vi "RES Build RES Table.vi"(8 "error in (no error)":errorcluster, 9 "Test Types 2":refnum<vi>, 10 "Message Queues in":T1, 11 "Settings in":T2={"Support"={"Save Configuration"={"Log File Base Path"=path "", "TDMS File Reference"=refnum, "Reset"=FALSE, "Wait"=0.0, "Start Time"=0.0, "Update Rate"=0, "Channel Names"=[], "System Preset"=variant}, "LOG Configuration"={"LOG REF"=refnum, "Writer Queue"=refnum, "Log Path"=path "", "LOG"=FALSE}, "ALARM Configuration"={"LOG REF"=refnum, "Writer Queue"=refnum, "Log Path"=path "", "UPS standby"=FALSE, "status code"=0, "SP"=[], "Over Sens Status"=[]}, "User Details"=[], "Radome Type"="", "Timer Configuration"={"Wait"=0.0, "Next Step"="", "Writer Queue"=refnum, "Reset"=FALSE, "VISA resource"="", "Status"=[], "Valve Time"=[], "Timer queue"=refnum, "Current valve"=0, "Enable"=FALSE}}, "Process"={"Test Configuration"={"current Step"=0, "Wait"=0.0, "Next Step"="", "Writer Queue"=refnum, "Reset"=FALSE, "SEQ Time"=0, "General Reset"=FALSE, "Cycles"=0, "Status"=[], "Ready"=[], "Backward"=FALSE, "Current SP"=[], "System Preset"={"Test Configuration"={"Cycles"=0, "Z Up"=0.0, "SP List"=[], "Operator"="", "Point Delay"=0, "Z Up 2"=0.0, "Cleaning In"=0.0, "Cleaning Out"=0.0, "Cleaning Cycles"=0}, "Test_Start_date"=""}, "Test Type"=enum."Calibration", "Sample Count"=0, "Local Queues"={"Cycles queue"=refnum, "Step queue"=refnum, "RES Queue"=refnum, "Clean queue"=refnum, "PS Scan queue"=refnum}, "current Clean"=0, "PS Measure Plan"=[]}}, "Report Configuration"={"Test Setting"={"Test_Num"=0, "Test_ID"=0, "Proc_ID"=0, "Max Force"=0.0, "User"="", "SN"="", "Date"=""}, "Measurements"=[], "LOG REF"=refnum, "Report Template"=path "", "Save Report path"=path "", "Data File Path"=path "", "Popup Dialog"=FALSE}, "History Data"={"Tests"=[], "Test Name"=""}, "Motor Configuration"={"Tango HW"={"VISA resource"="", "Baud Rate (115200)"=2, "lAnInterfaceType"=0, "bAShowProt"=15}, "Writer Queue"=refnum, "Status"=FALSE, "Abs Position"=[], "Axis Velocity"={"dX"=0.0, "dY"=0.0, "dZ"=0.0, "dA"=0.0}, "acceleration "=0.0, "Z direction"=enum."Up", "Position Mode"="", "plLSID"=0}, "PalmSense  Configuration"={"PalmSens.lvclass"=refnum, "Writer Queue"=refnum, "Enable"=FALSE, "Is Measuring Ref"=refnum, "Method"={"Name"="", "Method Ref"=variant}, "PS Live Curve Result"=refnum}, "Hiden Scanner Resources"={"Link"={"Connection"=enum."USB", "Host or IP address (TCP/IP)"="", "Port (Serial/USB)"="COM1"}, "VISA resource"="", "Writer Queue"=refnum, "Status"=FALSE}, "MFC Configuration"={"MFC Definition"={"MFC Port"="", "MFC Enable"=TRUE, "Baud Rate"=0, "Interface type"=enum."RS-485", "Address"=0}, "Set Point Options"={"Setpoint Value"=0.0, "Mass Flow EU 2"="", "Setpoint Source"="", "Valve Mode"=""}, "Writer Queue"=refnum, "Enable"=FALSE, "Update Rate"=0, "MRC Chamber Enable"=FALSE, "Selected Gas"="", "Address String"=""}} {"MFC Configuration"."Set Point Options"."Setpoint Value" min=0.0 max=0.62495 format="%.5f"; "Process"."Test Configuration"."PS Measure Plan" items=["Pretreatment settings (PS)", "Linear Sweep Voltammetry (LSV)", "Differential Pulse Voltammetry (DPV)", "Cyclic Voltammetry (CV)", "Chronoamperometry (CA)", "Chronopotentiometry (CP)", "El Imp Spectroscopy (EIS)"]; "Process"."Test Configuration"."System Preset"."Test Configuration"."SP List" format="%#.1g"; "Support"."Save Configuration"."Update Rate" min=1 max=10 step=1}) -> (0 "error out":errorcluster, 3 "Settings out 2":T2={"Support"={"Save Configuration"={"Log File Base Path"=path "", "TDMS File Reference"=refnum, "Reset"=FALSE, "Wait"=0.0, "Start Time"=0.0, "Update Rate"=0, "Channel Names"=[], "System Preset"=variant}, "LOG Configuration"={"LOG REF"=refnum, "Writer Queue"=refnum, "Log Path"=path "", "LOG"=FALSE}, "ALARM Configuration"={"LOG REF"=refnum, "Writer Queue"=refnum, "Log Path"=path "", "UPS standby"=FALSE, "status code"=0, "SP"=[], "Over Sens Status"=[]}, "User Details"=[], "Radome Type"="", "Timer Configuration"={"Wait"=0.0, "Next Step"="", "Writer Queue"=refnum, "Reset"=FALSE, "VISA resource"="", "Status"=[], "Valve Time"=[], "Timer queue"=refnum, "Current valve"=0, "Enable"=FALSE}}, "Process"={"Test Configuration"={"current Step"=0, "Wait"=0.0, "Next Step"="", "Writer Queue"=refnum, "Reset"=FALSE, "SEQ Time"=0, "General Reset"=FALSE, "Cycles"=0, "Status"=[], "Ready"=[], "Backward"=FALSE, "Current SP"=[], "System Preset"={"Test Configuration"={"Cycles"=0, "Z Up"=0.0, "SP List"=[], "Operator"="", "Point Delay"=0, "Z Up 2"=0.0, "Cleaning In"=0.0, "Cleaning Out"=0.0, "Cleaning Cycles"=0}, "Test_Start_date"=""}, "Test Type"=enum."Calibration", "Sample Count"=0, "Local Queues"={"Cycles queue"=refnum, "Step queue"=refnum, "RES Queue"=refnum, "Clean queue"=refnum, "PS Scan queue"=refnum}, "current Clean"=0, "PS Measure Plan"=[]}}, "Report Configuration"={"Test Setting"={"Test_Num"=0, "Test_ID"=0, "Proc_ID"=0, "Max Force"=0.0, "User"="", "SN"="", "Date"=""}, "Measurements"=[], "LOG REF"=refnum, "Report Template"=path "", "Save Report path"=path "", "Data File Path"=path "", "Popup Dialog"=FALSE}, "History Data"={"Tests"=[], "Test Name"=""}, "Motor Configuration"={"Tango HW"={"VISA resource"="", "Baud Rate (115200)"=2, "lAnInterfaceType"=0, "bAShowProt"=15}, "Writer Queue"=refnum, "Status"=FALSE, "Abs Position"=[], "Axis Velocity"={"dX"=0.0, "dY"=0.0, "dZ"=0.0, "dA"=0.0}, "acceleration "=0.0, "Z direction"=enum."Up", "Position Mode"="", "plLSID"=0}, "PalmSense  Configuration"={"PalmSens.lvclass"=refnum, "Writer Queue"=refnum, "Enable"=FALSE, "Is Measuring Ref"=refnum, "Method"={"Name"="", "Method Ref"=variant}, "PS Live Curve Result"=refnum}, "Hiden Scanner Resources"={"Link"={"Connection"=enum."USB", "Host or IP address (TCP/IP)"="", "Port (Serial/USB)"="COM1"}, "VISA resource"="", "Writer Queue"=refnum, "Status"=FALSE}, "MFC Configuration"={"MFC Definition"={"MFC Port"="", "MFC Enable"=TRUE, "Baud Rate"=0, "Interface type"=enum."RS-485", "Address"=0}, "Set Point Options"={"Setpoint Value"=0.0, "Mass Flow EU 2"="", "Setpoint Source"="", "Valve Mode"=""}, "Writer Queue"=refnum, "Enable"=FALSE, "Update Rate"=0, "MRC Chamber Enable"=FALSE, "Selected Gas"="", "Address String"=""}} {"MFC Configuration"."Set Point Options"."Setpoint Value" min=0.0 max=0.62495 format="%.5f"; "Process"."Test Configuration"."PS Measure Plan" items=["Pretreatment settings (PS)", "Linear Sweep Voltammetry (LSV)", "Differential Pulse Voltammetry (DPV)", "Cyclic Voltammetry (CV)", "Chronoamperometry (CA)", "Chronopotentiometry (CP)", "El Imp Spectroscopy (EIS)"]; "Process"."Test Configuration"."System Preset"."Test Configuration"."SP List" format="%#.1g"; "Support"."Save Configuration"."Update Rate" min=1 max=10 step=1})   [LabVIEW 2020]
uses:
  Settings.ctl
  <instrlib>/PalmSens SDK for LabVIEW 5.10/PalmSens/PalmSens.lvclass
  Logging/Save Configuration.ctl
  LOG/LOG Configuration.ctl
  support/Message Queue/Message Cluster.ctl
  ALARM/ALARM Configuration.ctl
  Valve Control/AM Configuration.ctl
  Test Driver/Test Driver Configuration.ctl
  Test Driver/System Preset.ctl
  Test Driver/Test Type.ctl
  Report/REP Configuration.ctl
  Report/Test Setting.ctl
  MOTOR/PS Hardware Configuration.ctl
  DMM/PalmSense Hardware Configuration.ctl
  Hiden Scanner/Scanner Hardware Configuration.ctl
  MRC/MRC Configuration.ctl
  support/Message Queue/All Message Queues.ctl
  support/Message Queue/Message Queue.lvlib
  Logging/SAVE.lvlib
  LOG/LOG.lvlib
  ALARM/QCT ALARM.lvlib
  Report/Report.lvlib
  Settings.lvlib
  MOTOR/MOTOR.lvlib
  Test Driver/Test Driver.lvlib
  DMM/PalmSens.lvlib
  Valve Control/Valve Control.lvlib
  Hiden Scanner/Hiden Scanner.lvlib
  MRC/MRC Module.lvlib
panel:
  in  "Test Types":string(tree)
  # "X"
  # "Y"
  # "Cycles"
  # "Point Delay"
  # "Up"
  # "Down"
  # "Z Axes"
  # "#C"
  # "In"
  # "Out"
  # "Cleaning [sec]"
  # "X"
  # "Y"
  # "Cycles"
  # "Point Delay"
  # "Up"
  # "Down"
  # "Z Axes"
  # "#C"
  # "In"
  # "Out"
  # "Cleaning [sec]"
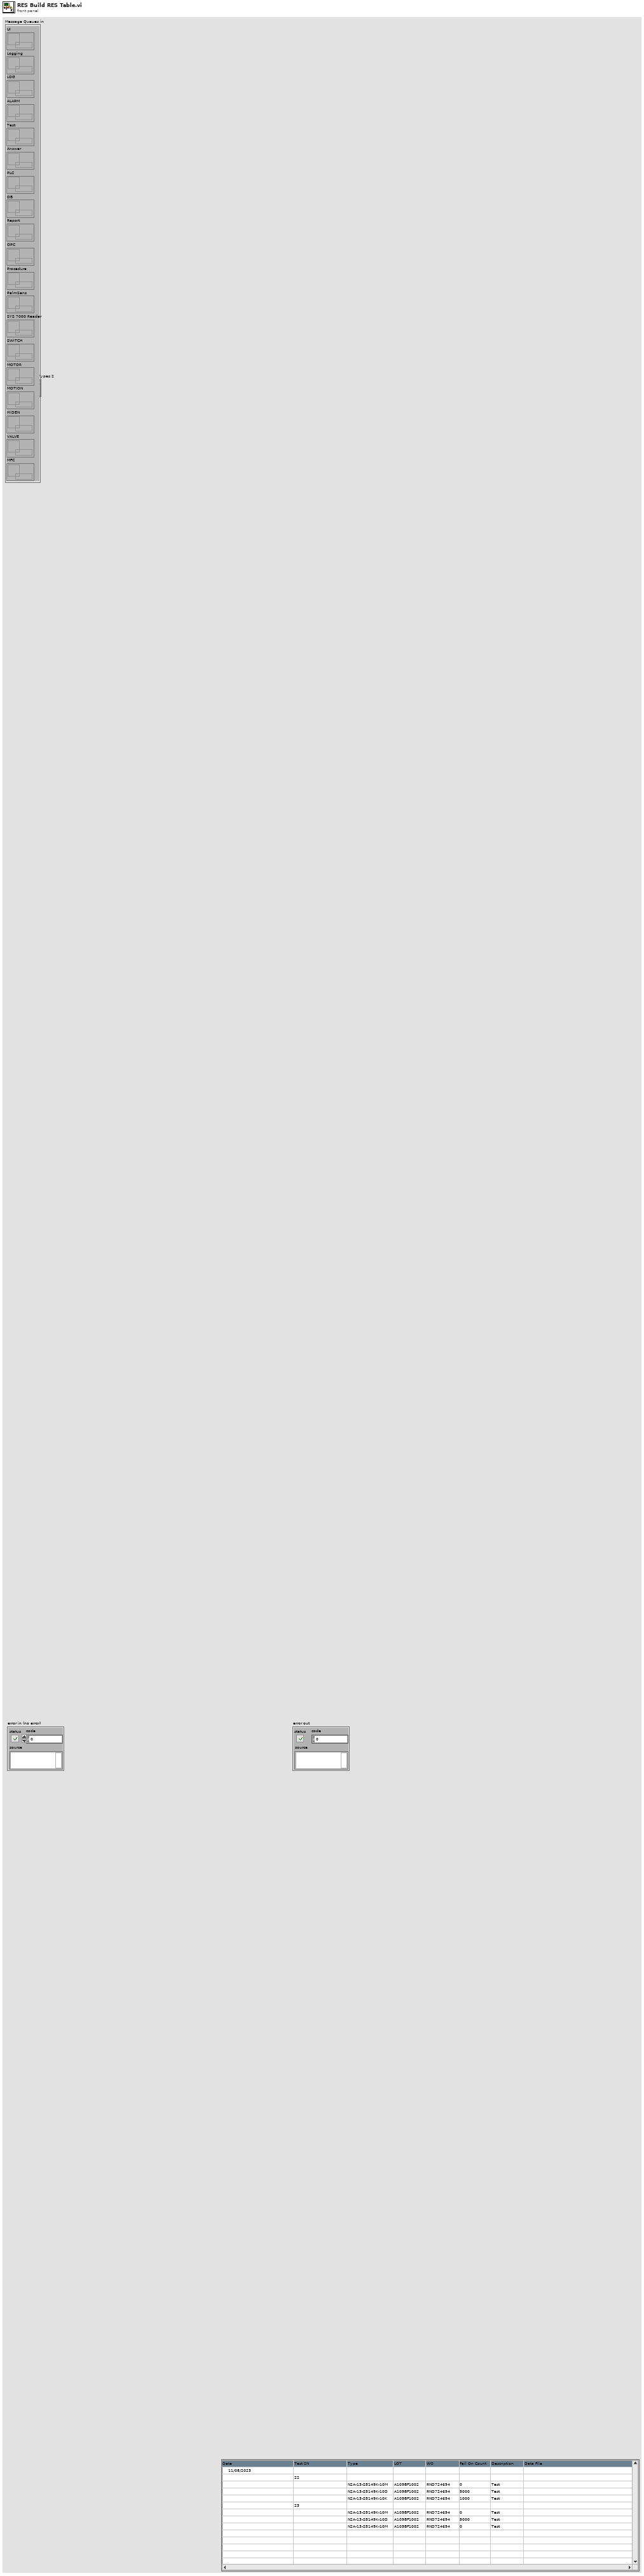
[diagram p1: front panel]
types:
  T1 = typedef "Message Queue.lvlib/All Message Queues.ctl" = cluster{"UI":refnum<queue>, "Logging":refnum<queue>, "LOG":refnum<queue>, "ALARM":refnum<queue>, "Test":refnum<queue>, "Answer":refnum<queue>, "PLC":refnum<queue>, "DB":refnum<queue>, "Report":refnum<queue>, "OPC":refnum<queue>, "Procedure":refnum<queue>, "PalmSens":refnum<queue>, "SYS 7000 Reader":refnum<queue>, "SWITCH":refnum<queue>, "MOTOR":refnum<queue>, "MOTION":refnum<queue>, "HIDEN":refnum<queue>, "VALVE":refnum<queue>, "MFC":refnum<queue>}
  T2 = typedef "Settings.lvlib/Settings.ctl" = cluster{"Support":cluster{"Save Configuration":T3, "LOG Configuration":T4, "ALARM Configuration":T5, "User Details":string[], "Radome Type":string, "Timer Configuration":T6}, "Process":cluster{"Test Configuration":T7}, "Report Configuration":T10, "History Data":cluster{"Tests":string[][], "Test Name":string}, "Motor Configuration":T12, "PalmSense  Configuration":T13, "Hiden Scanner Resources":T14, "MFC Configuration":T15}
  T3 = typedef "SAVE.lvlib/Save Configuration.ctl" = cluster{"Log File Base Path":path, "TDMS File Reference":refnum<k34>, "Reset":bool, "Wait":dbl, "Start Time":dbl, "Update Rate":u16, "Channel Names":string[], "System Preset":variant}
  T4 = typedef "LOG.lvlib/LOG Configuration.ctl" = cluster{"LOG REF":refnum<vi>, "Writer Queue":refnum<queue>, "Log Path":path, "LOG":bool}
  T5 = typedef "QCT ALARM.lvlib/ALARM Configuration.ctl" = cluster{"LOG REF":refnum<vi>, "Writer Queue":refnum<queue>, "Log Path":path, "UPS standby":bool, "status code":i32, "SP":dbl[], "Over Sens Status":dbl[]}
  T6 = typedef "Valve Control.lvlib/AM Configuration.ctl" = cluster{"Wait":dbl, "Next Step":string, "Writer Queue":refnum<queue>, "Reset":bool, "VISA resource":refnum<visa-resource-name>, "Status":bool[], "Valve Time":dbl[], "Timer queue":refnum<queue>, "Current valve":i32, "Enable":bool}
  T7 = typedef "Test Driver.lvlib/Test Driver Configuration.ctl" = cluster{"current Step":i32, "Wait":dbl, "Next Step":string, "Writer Queue":refnum<queue>, "Reset":bool, "SEQ Time":i32, "General Reset":bool, "Cycles":i32, "Status":bool[], "Ready":bool[], "Backward":bool, "Current SP":dbl[], "System Preset":T8, "Test Type":T9, "Sample Count":i32, "Local Queues":cluster{"Cycles queue":refnum<queue>, "Step queue":refnum<queue>, "RES Queue":refnum<queue>, "Clean queue":refnum<queue>, "PS Scan queue":refnum<queue>}, "current Clean":i32, "PS Measure Plan":u16[]}
  T8 = typedef "System Preset.ctl" = cluster{"Test Configuration":cluster{"Cycles":i32, "Z Up":dbl, "SP List":dbl[][], "Operator":string, "Point Delay":i32, "Z Up 2":dbl, "Cleaning In":dbl, "Cleaning Out":dbl, "Cleaning Cycles":i32}, "Test_Start_date":string}
  T9 = typedef "Test Driver.lvlib/Test Type.ctl" = enum16{"Calibration", "Test"}
  T10 = typedef "Report.lvlib/REP Configuration.ctl" = cluster{"Test Setting":T11, "Measurements":string[][], "LOG REF":refnum<vi>, "Report Template":path, "Save Report path":path, "Data File Path":path, "Popup Dialog":bool}
  T11 = typedef "Report.lvlib/Test Setting.ctl" = cluster{"Test_Num":i32, "Test_ID":i32, "Proc_ID":i32, "Max Force":dbl, "User":string, "SN":string, "Date":string}
  T12 = typedef "MOTOR.lvlib/PS Hardware Configuration.ctl" = cluster{"Tango HW":cluster{"VISA resource":refnum<visa-resource-name>, "Baud Rate (115200)":i32, "lAnInterfaceType":i32, "bAShowProt":i32}, "Writer Queue":refnum<queue>, "Status":bool, "Abs Position":i32[], "Axis Velocity":cluster{"dX":dbl, "dY":dbl, "dZ":dbl, "dA":dbl}, "acceleration ":dbl, "Z direction":enum16{"Up", "Down"}, "Position Mode":string, "plLSID":i32}
  T13 = typedef "PalmSens.lvlib/PalmSense Hardware Configuration.ctl" = cluster{"PalmSens.lvclass":refnum<class "PalmSens.lvclass">, "Writer Queue":refnum<queue>, "Enable":bool, "Is Measuring Ref":refnum<vi>, "Method":cluster{"Name":string, "Method Ref":variant}, "PS Live Curve Result":refnum<vi>}
  T14 = typedef "Hiden Scanner.lvlib/Scanner Hardware Configuration.ctl" = cluster{"Link":cluster{"Connection":enum16{"Serial", "TCP/IP", "USB"}, "Host or IP address (TCP/IP)":string, "Port (Serial/USB)":string}, "VISA resource":refnum<visa-resource-name>, "Writer Queue":refnum<queue>, "Status":bool}
  T15 = typedef "MRC Module.lvlib/MRC Configuration.ctl" = cluster{"MFC Definition":cluster{"MFC Port":refnum<visa-resource-name>, "MFC Enable":bool, "Baud Rate":i32, "Interface type":enum32{"RS-485", "RS-232"}, "Address":i32}, "Set Point Options":cluster{"Setpoint Value":dbl, "Mass Flow EU 2":string, "Setpoint Source":string, "Valve Mode":string}, "Writer Queue":refnum<queue>, "Enable":bool, "Update Rate":u32, "MRC Chamber Enable":bool, "Selected Gas":string, "Address String":string}
  T16 = cluster{"Type CMD":string, "Mode CMD":string, "Main CMD":string}
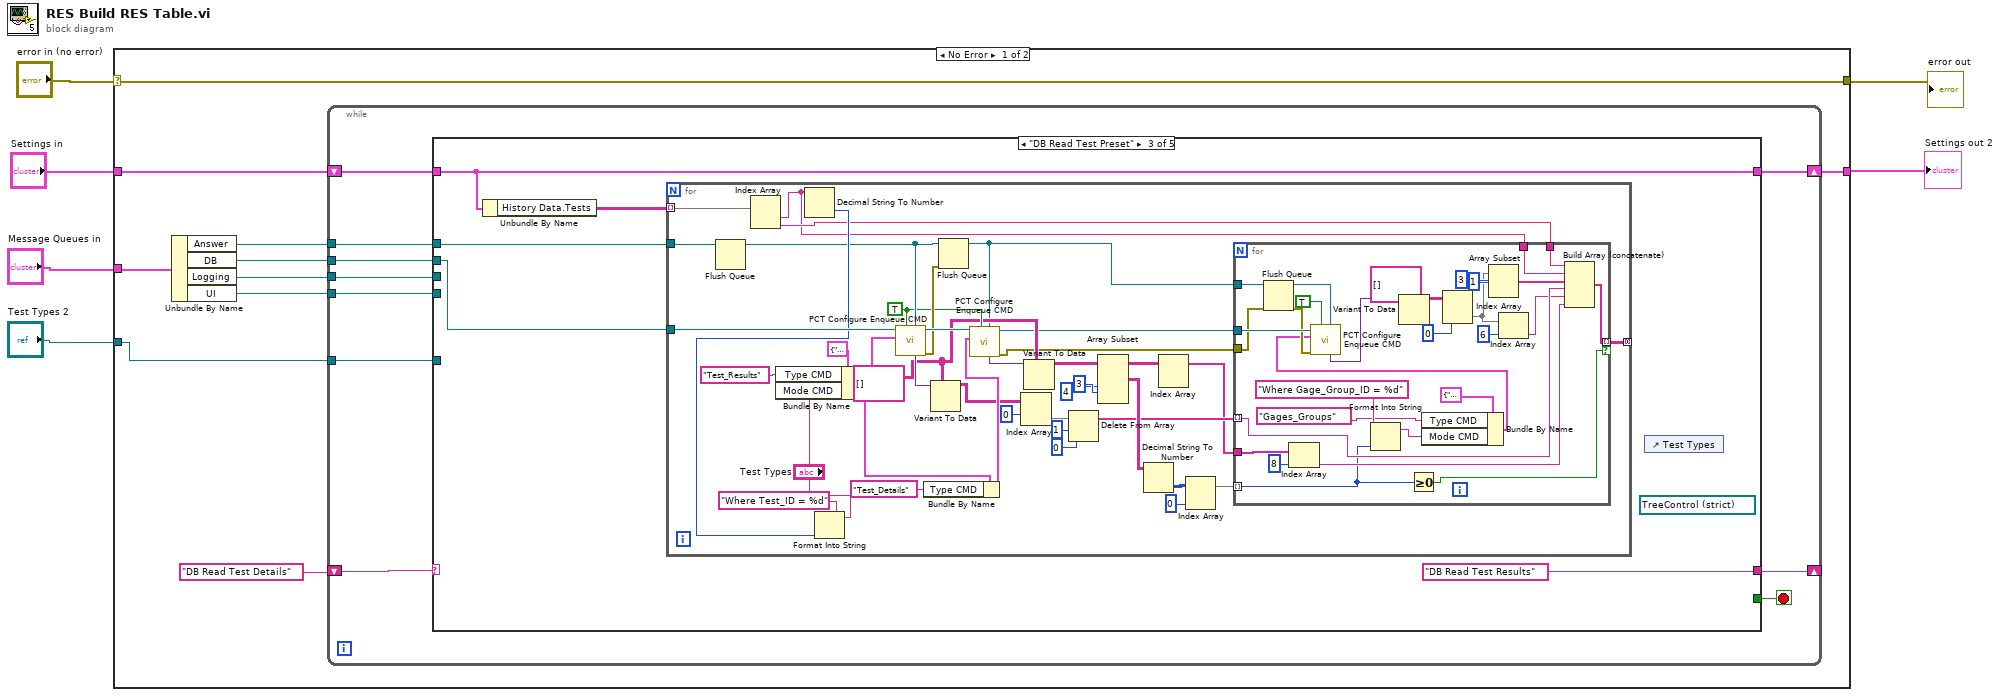
[diagram p0: block diagram]
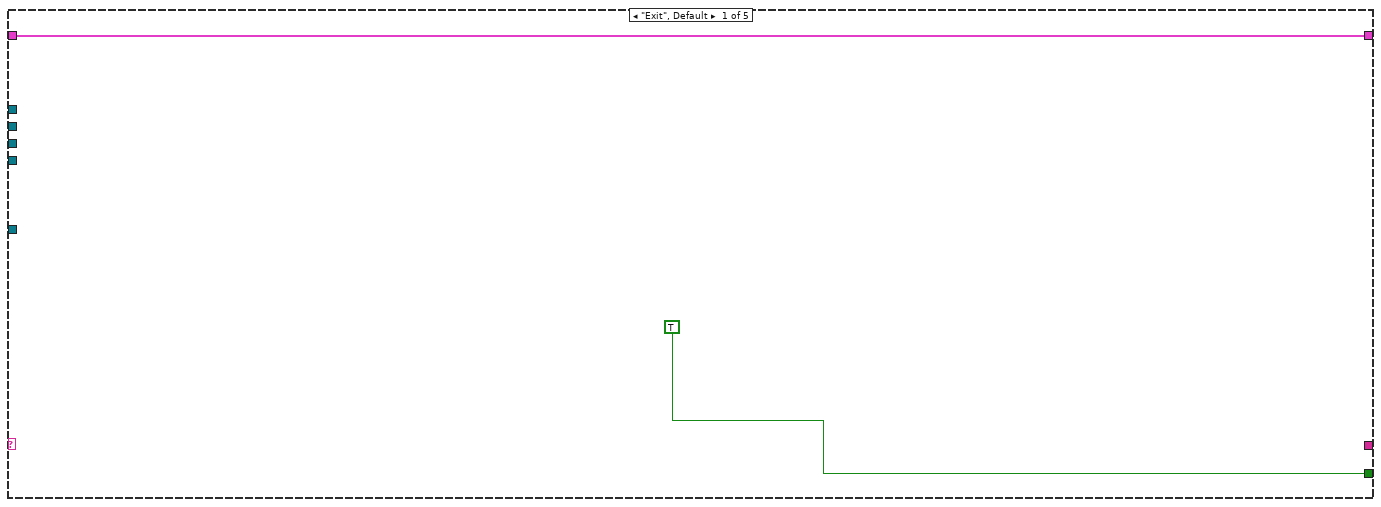
[diagram p2: hidden frame]
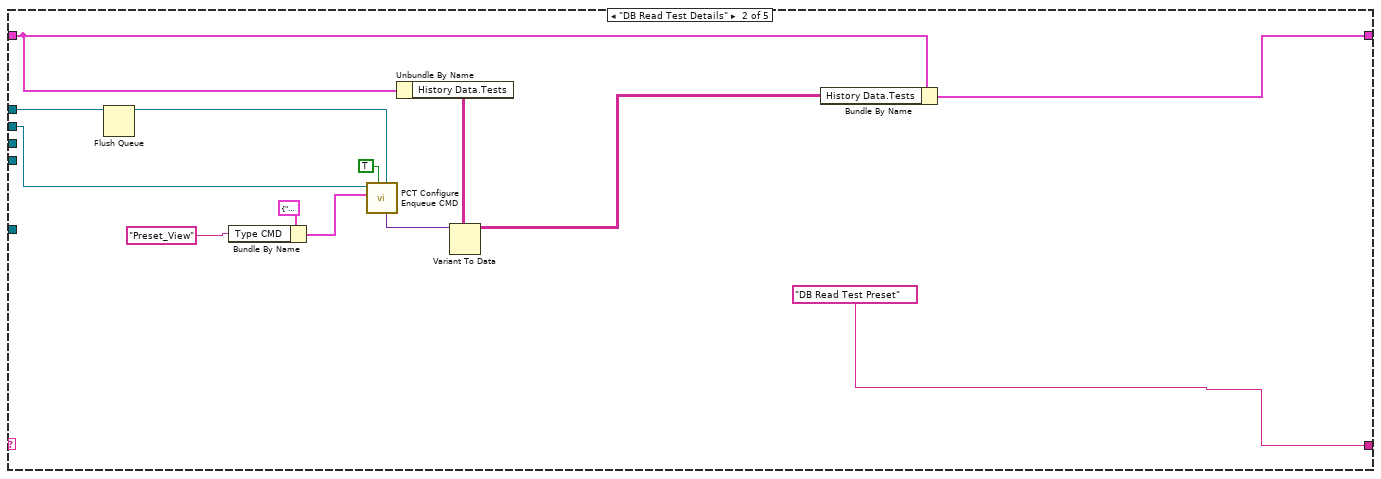
[diagram p3: hidden frame]
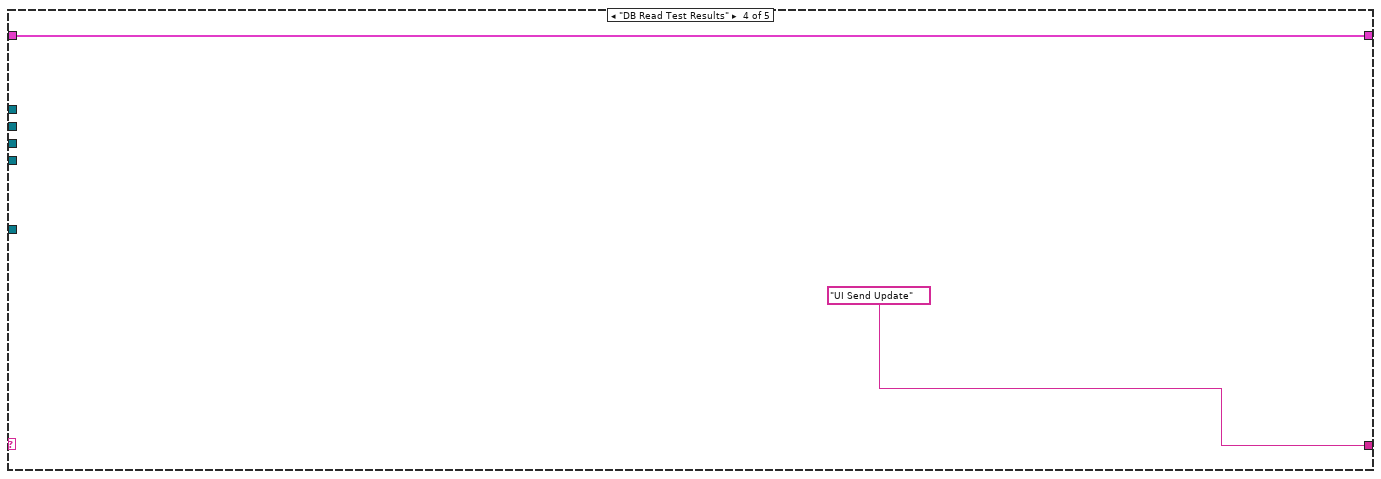
[diagram p4: hidden frame]
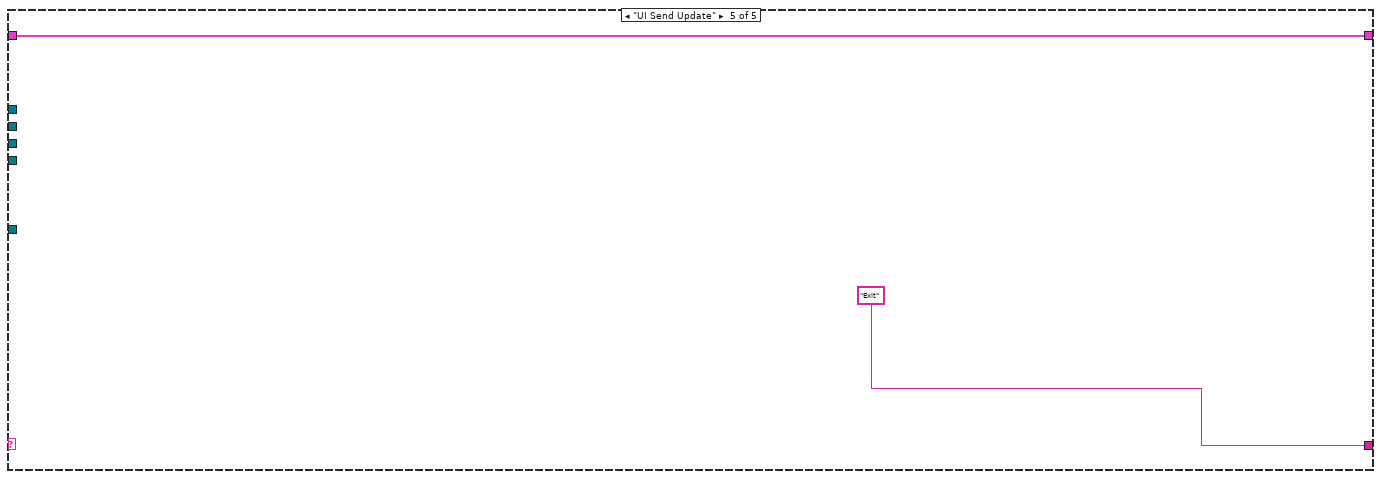
[diagram p5: hidden frame]
diagram:
  n1 = case shown="No Error" "error in (no error)" {
    selector: "error in (no error)" -> [w16 w120]
    tunnel: [w16 w120] -> w1
    tunnel: "Message Queues in" -> [w11 _]
    tunnel: "Test Types 2" -> [w7 _]
    tunnel: "Settings in" -> [w9 w119]
    tunnel: [w8 w119] -> w4
    frame No Error {
      n2 = Unbundle By Name(w11) -> ("Answer"=w13:refnum<queue>, "DB"=w14:refnum<queue>, "Logging"=w12:refnum<queue>, "UI"=w15:refnum<queue>)
      n3 = while {
        shift-right: [w24] -> _
        shift-left: "DB Read Test Details" ("CMD") -> [w26]
        tunnel: w7 -> [w25]
        shift-right: [w21] -> w8
        shift-left: w9 -> [w23]
        tunnel: w12 -> [w22]
        tunnel: w13 -> [w20]
        tunnel: w14 -> [w19]
        tunnel: w15 -> [w18]
        stop <- w17 stop-if-true
        n4 = case shown="\"DB Read Test Preset\"" w26 {
          tunnel: w25 -> [_ _ _ _ _]
          tunnel: [_ "DB Read Test Preset" ("CMD") "DB Read Test Results" ("CMD") "UI Send Update" ("CMD") "Exit" ("CMD")] -> w24
          tunnel: w23 -> [w28 w32 w45 w115 w118]
          tunnel: w22 -> [_ _ _ _ _]
          tunnel: [w28 w31 w45 w115 w118] -> w21
          tunnel: w20 -> [_ w36 w44 _ _]
          tunnel: w19 -> [_ w37 w43 _ _]
          tunnel: w18 -> [_ _ _ _ _]
          tunnel: [TRUE _ _ _ _] -> w17
          frame "Exit", Default {
          }
          frame "DB Read Test Details" {
            n5 = Flush Queue(queue=w36) -> (queue out=w35:refnum<queue>)  [unwired: 1 in, 2 out]
            n6 = Bundle By Name(cluster=T16 {"Type CMD"="Test_Count", "Mode CMD"="", "Main CMD"="Get Data"} ("CMD"), "Type CMD"="Preset_View") -> (w40:T16)
            n7 = call "PCT Configure Enqueue CMD.vi"("Response Queue"=w35, "Read"=TRUE, "CMD"=w40, "CMD Queue in"=w37) -> ("Message Data"=w33:variant)  [unwired: 5 in, 2 out]
            n8 = Unbundle By Name(w32) -> ("History Data.Tests"=w29:string[][])
            n9 = Variant To Data(type=w29, Variant=w33) -> (data=w30:string[][])  [unwired: 1 in, 1 out]
            n10 = Bundle By Name(cluster=w32, "History Data.Tests"=w30) -> (w31:T2)
          }
          frame "DB Read Test Preset" {
            (unwired) refnum<vi> refnum ("Test Types")
            n11 = Unbundle By Name(w45) -> ("History Data.Tests"=w42:string[][])
            n12 = for {
              tunnel: w44 -> [w81]
              tunnel: w43 -> [w80]
              tunnel: w42 -> [w79] mode=indexing
              tunnel: [w56] -> _ mode=concatenating
              w68 = string[][] [] ("Gages Group")
              w72 = TRUE ("Read")
              n13 = Flush Queue(queue=w81) -> (queue out=w73:refnum<queue>)  [unwired: 1 in, 2 out]
              n14 = Index Array(array=w79) -> (element #1=w47:string, element #2=w57:string)  [unwired: 2 in]
              n15 = Decimal String To Number(string=w47) -> (number=w77:i32)  [unwired: 2 in, 1 out]
              n16 = Format Into String(format string="Where Test_ID = %d" ("Type CMD"), w77) -> (resulting string=w76:string)  [unwired: 2 in, 1 out]
              n17 = Bundle By Name(cluster=T16 {"Type CMD"="Test_Count", "Mode CMD"="", "Main CMD"="Get Data"} ("CMD"), "Type CMD"="Test_Results", "Mode CMD"=w76) -> (w71:T16)
              n18 = call "PCT Configure Enqueue CMD.vi"("Response Queue"=w73, "Read"=w72, "CMD"=w71, "CMD Queue in"=w80) -> ("error out"=w74:errorcluster, "CMD Queue out"=w75:refnum<queue>, "Message Data"=w82:variant)  [unwired: 5 in]
              n19 = Bundle By Name(cluster=w71, "Type CMD"="Test_Details") -> (w70:T16)
              n20 = Variant To Data(type=w68, Variant=w82) -> (data=w58:string[][])  [unwired: 1 in, 1 out]
              n21 = Flush Queue(queue=w73, error in (no error)=w74) -> (queue out=w59:refnum<queue>)  [unwired: 2 out]
              n22 = call "PCT Configure Enqueue CMD.vi"("Response Queue"=w59, "Read"=w72, "CMD"=w70, "CMD Queue in"=w75) -> ("error out"=w60:errorcluster, "CMD Queue out"=w61:refnum<queue>, "Message Data"=w67:variant)  [unwired: 5 in]
              n23 = Index Array(array=w58, index (row)=0) -> (element=w51:string[])  [unwired: 1 in]
              n24 = Variant To Data(type=w68, Variant=w67) -> (data=w49:string[][])  [unwired: 1 in, 1 out]
              n25 = Delete From Array(array=w51, length=1, index=0) -> (array with subset deleted=w50:string[])  [unwired: 1 out]
              n26 = Array Subset(array=w49, index (col)=3 ("index"), length (col)=4 ("length")) -> (w55:string[][])  [unwired: 2 in]
              n27 = Decimal String To Number(string=w55) -> (number=w64:i32[][])  [unwired: 2 in, 1 out]
              n28 = Index Array(array=w49) -> (element=w48:string[])  [unwired: 2 in]
              n29 = Index Array(array=w64, index (row)=0) -> (element=w63:i32[])  [unwired: 1 in]
              n30 = for {
                tunnel: w63 -> [w91] mode=indexing
                tunnel: w61 -> [w114]
                tunnel: w60 -> [w113]
                tunnel: w59 -> [w111]
                tunnel: w50 -> [w97] mode=indexing
                tunnel: w57 -> [w89]
                tunnel: [w96] -> w56 mode=indexing if=w90
                tunnel: w48 -> [w95]
                tunnel: w47 -> [w88]
                n31 = Flush Queue(queue=w111, error in (no error)=w113) -> (queue out=w110:refnum<queue>, error out=w112:errorcluster)  [unwired: 1 out]
                n32 = Index Array(array=w95, index=8) -> (element=w93:string)
                n33 = Format Into String(format string="Where Gage_Group_ID = %d" ("Type CMD"), w91) -> (resulting string=w107:string)  [unwired: 2 in, 1 out]
                n34 = Greater Or Equal To 0?(x=w91) -> (x >= 0?=w90:bool)
                n35 = Bundle By Name(cluster=T16 {"Type CMD"="Test_Count", "Mode CMD"="", "Main CMD"="Get Data"} ("CMD"), "Type CMD"="Gages_Groups" ("CMD"), "Mode CMD"=w107) -> (w92:T16)
                n36 = call "PCT Configure Enqueue CMD.vi"("Response Queue"=w110, "Read"=TRUE, "error in (no error)"=w112, "CMD"=w92, "CMD Queue in"=w114) -> ("Message Data"=w104:variant)  [unwired: 4 in, 2 out]
                n37 = Variant To Data(type=string[][] [] ("Gages Group"), Variant=w104) -> (data=w102:string[][])  [unwired: 1 in, 1 out]
                n38 = Index Array(array=w102, index (row)=0) -> (element=w87:string[])  [unwired: 1 in]
                n39 = Array Subset(array=w87, index=1, length=3) -> (w98:string[])
                n40 = Index Array(array=w87, index=6) -> (element=w86:string)
                n41 = Build Array (concatenate)(w89, w88, w98, w97, w86, w93) -> (w96:string[])
              }
            }
            n42 = control-ref of="Test Types"() -> ()  [unwired: 1 out]
          }
          frame "DB Read Test Results" {
          }
          frame "UI Send Update" {
          }
        }
      }
    }
    frame Error {
    }
  }
  "Settings out 2" <- w4
  "error out" <- w1
